vi "array_extract_positive.vi"(1 "input":i32[](array[numeric])) -> (0 "output":i32[](array[numeric]))   [LabVIEW 2020]
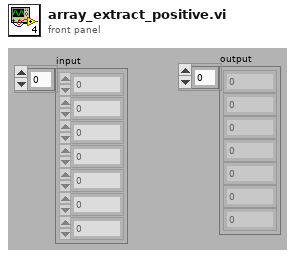
[diagram p1: front panel]
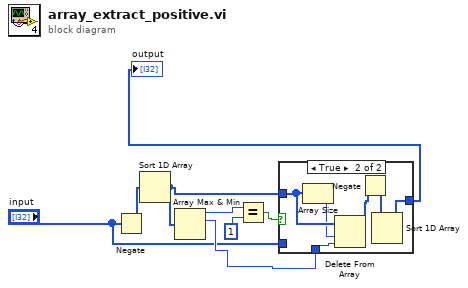
[diagram p0: block diagram]
diagram:
  n1 = Negate(x="input") -> (-x=w7:i32[])
  n2 = Sort 1D Array(array=w7) -> (sorted array=w6:i32[])
  n3 = Array Max & Min(array=w6) -> (max value=w1:i32, max index (indices)=w5:i32)  [unwired: 2 out]
  n4 = Equal?(x=w1, y=1) -> (x = y?=w3:bool)
  n5 = case shown="True" w3 {
    tunnel: "input" -> [w9 _]
    tunnel: [w9 w11] -> w8
    tunnel: w6 -> [_ w15]
    tunnel: w5 -> [_ w13]
    frame False {
    }
    frame True {
      n6 = Array Size(array=w15) -> (size(s)=w14:i32)
      n7 = Delete From Array(array=w15, length=w14, index=w13) -> (array with subset deleted=w12:i32[])  [unwired: 1 out]
      n8 = Negate(x=w12) -> (-x=w10:i32[])
      n9 = Sort 1D Array(array=w10) -> (sorted array=w11:i32[])
    }
  }
  "output" <- w8
